vi "SequencedStructure.vi"() -> ()   [LabVIEW 2019]
panel:
  in  "stop 2":bool
  out "Waveform Chart 2":dbl(graph)
  out "Waveform Chart":dbl(graph)
  in  "stop":bool
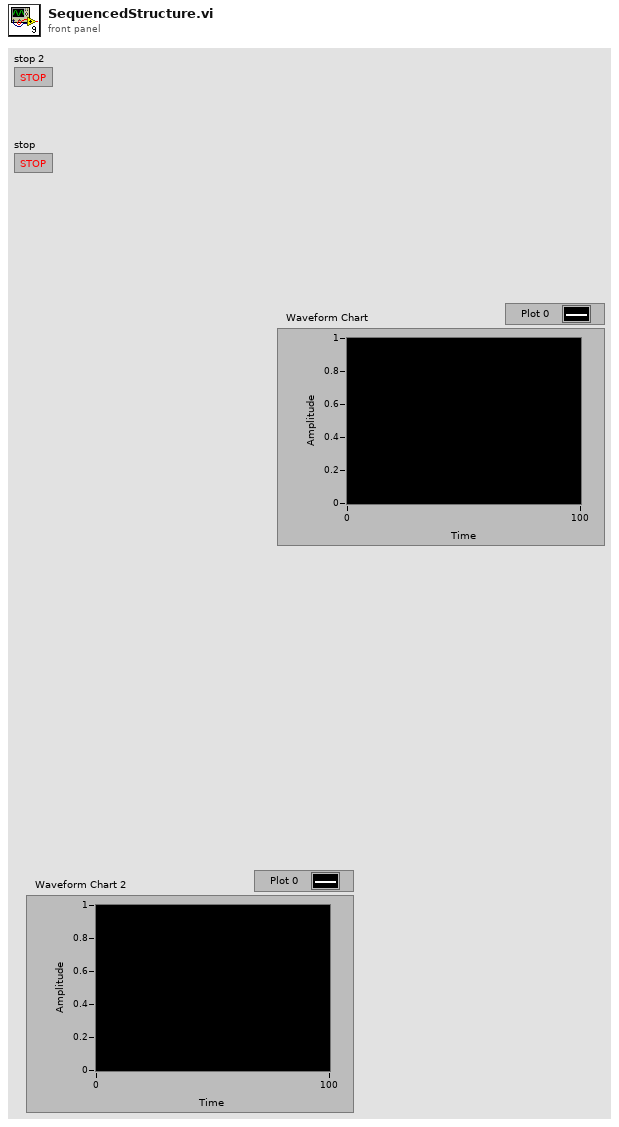
[diagram p1: front panel]
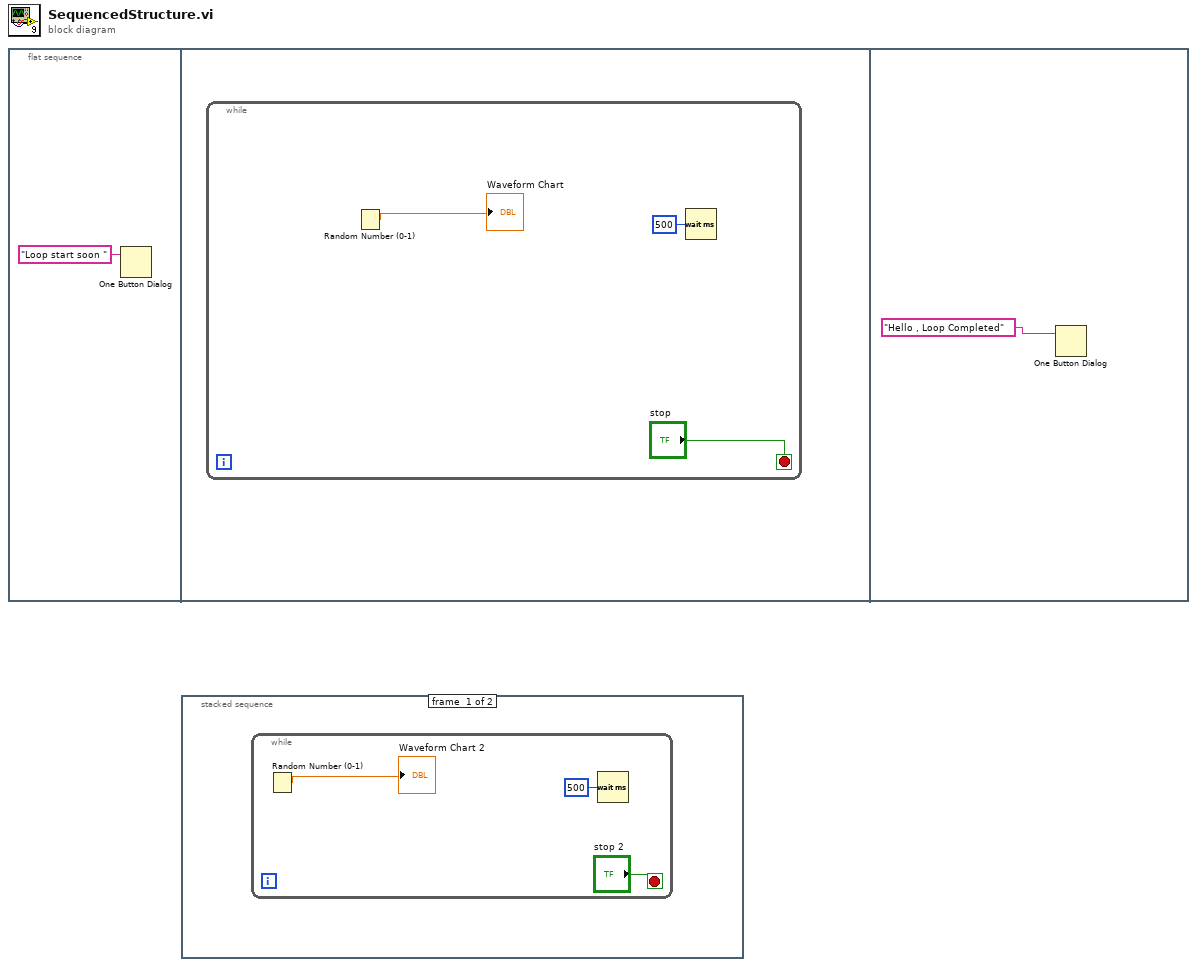
[diagram p0: block diagram]
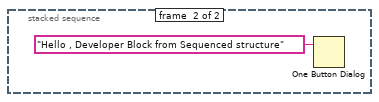
[diagram p2: hidden frame]
diagram:
  n1 = flat-sequence {
    frame #0 {
      n2 = One Button Dialog(message="Loop start soon ") -> ()  [unwired: 1 in, 1 out]
    }
    frame #1 {
      n3 = while {
        stop <- "stop" stop-if-true
        n4 = Random Number (0-1)() -> (number: 0 to 1=→"Waveform Chart":dbl)
        n5 = Wait (ms)(milliseconds to wait=u32 500) -> ()  [unwired: 1 out]
      }
    }
    frame #2 {
      n6 = One Button Dialog(message="Hello , Loop Completed") -> ()  [unwired: 1 in, 1 out]
    }
  }
  n7 = stacked-sequence {
    frame #0 {
      n8 = while {
        stop <- "stop 2" stop-if-true
        n9 = Random Number (0-1)() -> (number: 0 to 1=→"Waveform Chart 2":dbl)
        n10 = Wait (ms)(milliseconds to wait=u32 500) -> ()  [unwired: 1 out]
      }
    }
    frame #1 {
      n11 = One Button Dialog(message="Hello , Developer Block from Sequenced structure") -> ()  [unwired: 1 in, 1 out]
    }
  }
